vi "Reset all pane origins.vi"(8 "error in (no error":errorcluster, 11 "Vi Ref In":refnum<vi>) -> (0 "error out":errorcluster, 3 "Vi Ref Out":refnum<vi>)   [LabVIEW 2012, in "GUI.lvlib"]
doc: "Resets all panes to 0,0 origin from the referenced vi."
uses:
  GUI.lvlib
  <vilib>/Utility/miscctls.llb/LVPointTypeDef.ctl
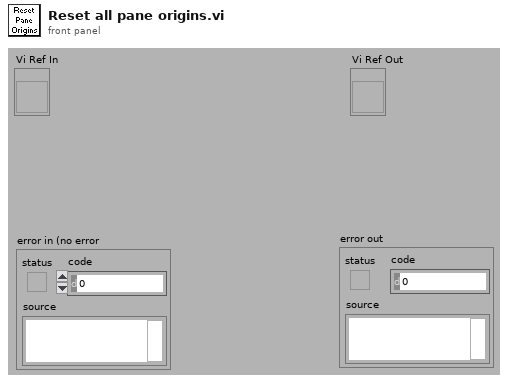
[diagram p1: front panel]
types:
  T1 = typedef "LVPointTypeDef.ctl" = cluster{"Horizontal":i16, "Vertical":i16}
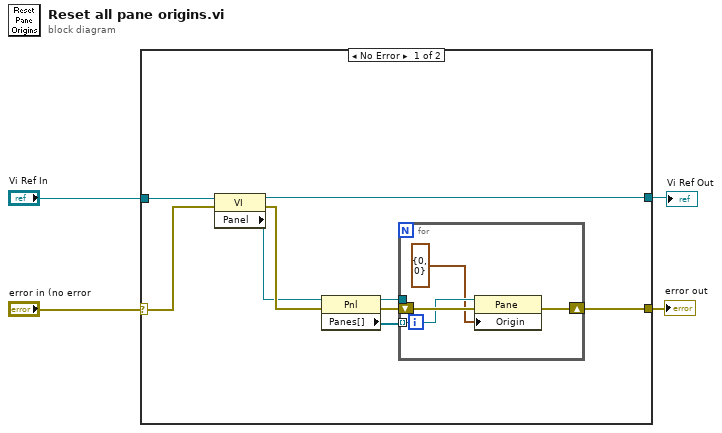
[diagram p0: block diagram]
diagram:
  n1 = case shown="No Error" "error in (no error" {
    selector: "error in (no error" -> [w6 w19]
    tunnel: [w13 w19] -> w4
    tunnel: "Vi Ref In" -> [w7 w18]
    tunnel: [w5 w18] -> w1
    frame No Error {
      n2 = property class="VI"(reference=w7, error in=w6) -> (reference out=w5:refnum<vi>, error out=w9:errorcluster, "Panel"=w8:refnum<vi>)
      n3 = property class="Pnl"(reference=w8, error in=w9) -> (reference out=w11:refnum<vi>, error out=w10:errorcluster, "Panes[]"=w12:refnum<vi>[])
      n4 = for {
        tunnel: w11 -> [_]
        tunnel: w12 -> [w16] mode=indexing
        shift-right: [w15] -> w13
        shift-left: w10 -> [w17]
        n5 = property class="Pane"(reference=w16, error in=w17, "Origin"=T1 {"Horizontal"=0, "Vertical"=0}) -> (error out=w15:errorcluster)  [unwired: 1 out]
      }
    }
    frame Error {
    }
  }
  "error out" <- w4
  "Vi Ref Out" <- w1
